vi "Configure Frequency.vi"(7 "Mode":enum16{"Center Span", "Start Stop"}(ring), 8 "error in (no error)":errorcluster, 9 "Span/Stop Frequency":dbl, 10 "Center/Start Frequency":dbl, 11 "Vector Network Analyzer in":refnum<class "Vector Network Analyzer.lvclass">) -> (0 "error out":errorcluster, 3 "Vector Network Analyzer out":refnum<class "Vector Network Analyzer.lvclass">)   [LabVIEW 2020, in "Vector Network Analyzer.lvclass"]
doc: "Configures the frequency range for the sweep.\nThe default mode is Center Span."
uses:
  Vector Network Analyzer.lvclass
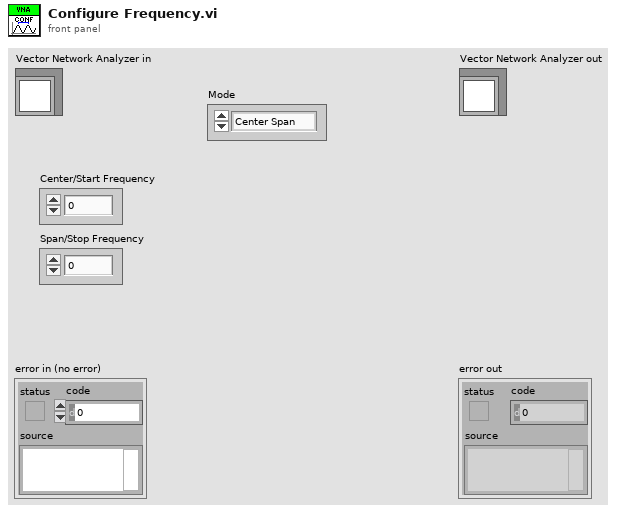
[diagram p1: front panel]
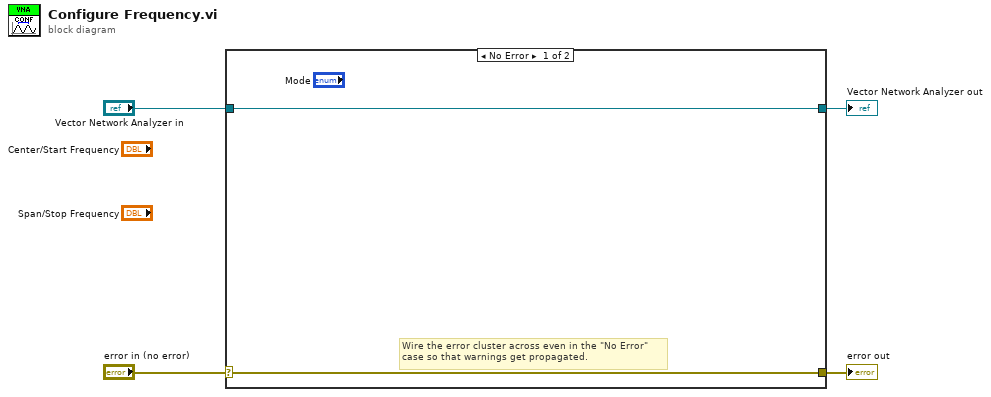
[diagram p0: block diagram]
diagram:
  n1 = case shown="No Error" "error in (no error)" {
    selector: "error in (no error)" -> [w5 w8]
    tunnel: [w5 w8] -> w3
    tunnel: [w6 w7] -> w1
    tunnel: "Vector Network Analyzer in" -> [w6 w7]
    frame No Error {
      # "Wire the error cluster across even in the \"No Error\"\ncase so that warnings get propagated."
    }
    frame Error {
    }
  }
  "error out" <- w3
  "Vector Network Analyzer out" <- w1
